vi "WLM0.vi"(1 "In":variant, 2 "Mode":u32(ring) items=["Open", "Close", "Begin", "End", "Get", "Set"]) -> (0 "Out":variant)   [LabVIEW 2014]
uses:
  wlmData.dll
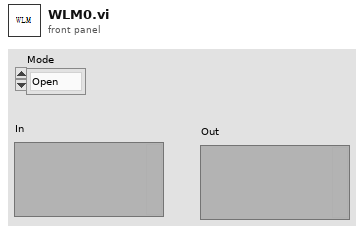
[diagram p1: front panel]
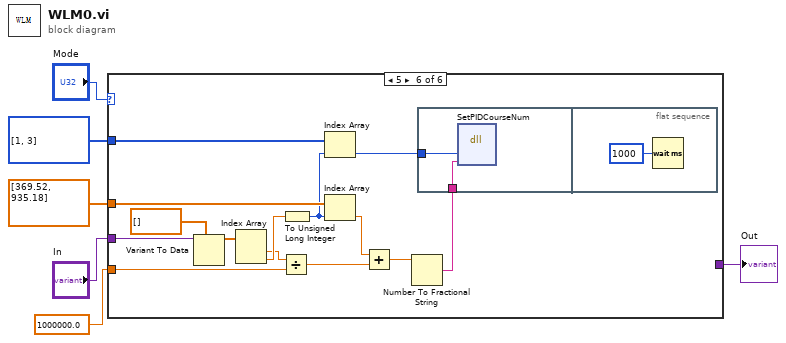
[diagram p0: block diagram]
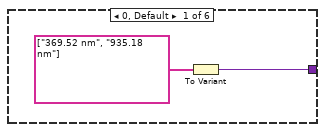
[diagram p2: hidden frame]
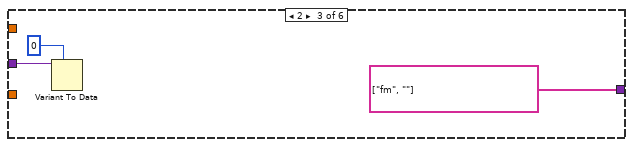
[diagram p4: hidden frame]
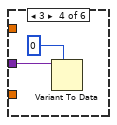
[diagram p5: hidden frame]
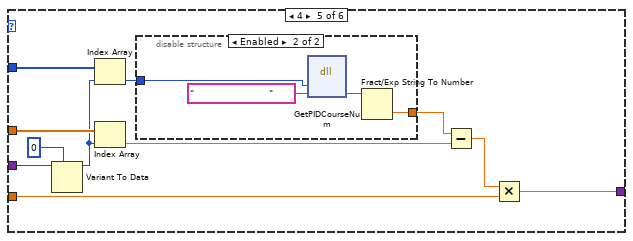
[diagram p6: hidden frame]
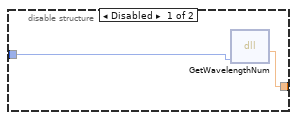
[diagram p7: hidden frame]
diagram:
  n1 = case shown="5" "Mode" {
    tunnel: "In" -> [_ _ w11 w12 w23 w43]
    tunnel: [w7 _ string[] ["fm", ""] ("Strings []") _ w15 _] -> w4
    tunnel: u32[] [1, 3] -> [_ _ _ _ w22 w35]
    tunnel: dbl[] [369.52, 935.18] -> [_ _ _ _ w19 w38]
    tunnel: 1000000.0 ("y") -> [_ _ _ _ w14 w39]
    frame 0, Default {
      n2 = To Variant(anything=string[] ["369.52 nm", "935.18 nm"] ("Strings []")) -> (Variant=w7:variant)
    }
    frame 1 {
    }
    frame 2 {
      n3 = Variant To Data(type=0, Variant=w11) -> ()  [unwired: 1 in, 2 out]
    }
    frame 3 {
      n4 = Variant To Data(type=0, Variant=w12) -> ()  [unwired: 1 in, 2 out]
    }
    frame 4 {
      n5 = Variant To Data(type=u32 0, Variant=w23) -> (data=w18:u32)  [unwired: 1 in, 1 out]
      n6 = Index Array(array=w22, index=w18) -> (element=w21:u32)
      n7 = Index Array(array=w19, index=w18) -> (element=w17:dbl)
      n8 = disable-structure shown="Enabled" {
        disable-tunnel: w21 -> [w26 w30]
        disable-tunnel: [w25 w28] -> w20
        frame Disabled {
          n9 = dll-call lib="wlmData.dll" fn="GetWavelengthNum"("ch"=w26) -> ("wl"=w25:dbl)  [unwired: 4 in, 2 out]
        }
        frame Enabled {
          n10 = dll-call lib="wlmData.dll" fn="GetPIDCourseNum"("ch"=w30, "str"="                         ") -> ("str"=w29:string)  [unwired: 5 in, 2 out]
          n11 = Fract/Exp String To Number(string=w29) -> (number=w28:dbl)  [unwired: 3 in, 1 out]
        }
      }
      n12 = Subtract(x=w20, y=w17) -> (x-y=w16:dbl)
      n13 = Multiply(x=w16, y=w14) -> (x*y=w15:dbl)
    }
    frame 5 {
      n14 = Variant To Data(type=dbl[] [] ("appended array"), Variant=w43) -> (data=w42:dbl[])  [unwired: 1 in, 1 out]
      n15 = Index Array(array=w42) -> (element #1=w40:dbl, element #2=w41:dbl)  [unwired: 2 in]
      n16 = Divide(x=w40, y=w39) -> (x/y=w36:dbl)
      n17 = To Unsigned Long Integer(number=w41) -> (unsigned 32bit integer=w34:u32)
      n18 = Index Array(array=w35, index=w34) -> (element=w33:u32)
      n19 = Index Array(array=w38, index=w34) -> (element=w37:dbl)
      n20 = Add(x=w37, y=w36) -> (x+y=w32:dbl)
      n21 = Number To Fractional String(number=w32) -> (F-format string=w31:string)  [unwired: 3 in]
      n22 = flat-sequence {
        tunnel: w33 -> [w46]
        tunnel: w31 -> [w45]
        frame #0 {
          n23 = dll-call lib="wlmData.dll" fn="SetPIDCourseNum"("ch"=w46, "str"=w45) -> ()  [unwired: 6 in, 2 out]
        }
        frame #1 {
          n24 = Wait (ms)(milliseconds to wait=u32 1000) -> ()  [unwired: 1 out]
        }
      }
    }
  }
  "Out" <- w4
